vi "LV_call_transfer.vi"() -> ()   [LabVIEW 2020]
panel:
  out "return code":i32
  out "standard output":string
  out "error out":errorcluster
  out "Path to Python script":path
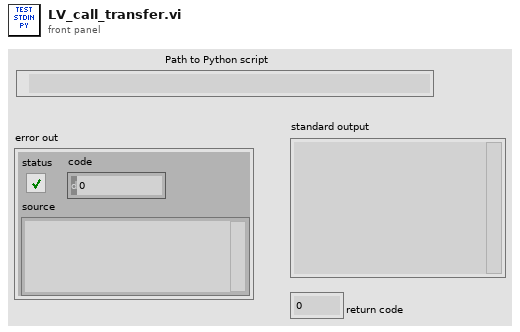
[diagram p1: front panel]
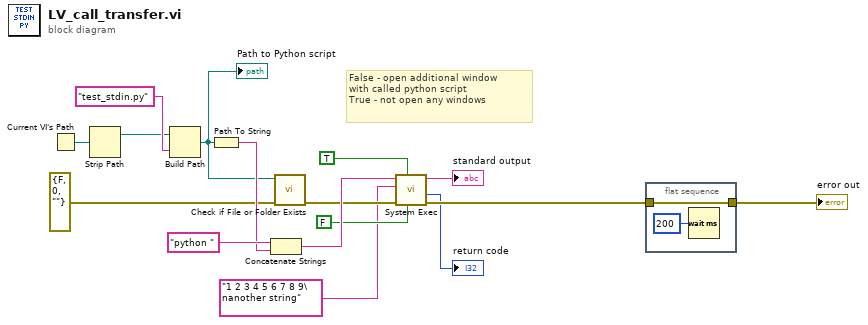
[diagram p0: block diagram]
diagram:
  # "False - open additional window\nwith called python script\nTrue - not open any windows"
  n1 = Current VI's Path() -> (path=w16:path)
  n2 = Strip Path(path=w16) -> (stripped path=w10:path)  [unwired: 1 out]
  n3 = Build Path(base path=w10, name or relative path="test_stdin.py" ("string")) -> (appended path=w8:path)
  "Path to Python script" <- w8
  n4 = Path To String(path=w8) -> (string=w11:string)
  n5 = Concatenate Strings("python " ("command line"), w11) -> (w14:string)
  n6 = call <vilib>:"Check if File or Folder Exists.vi"("error in (no error)"=errorcluster {"status"=FALSE, "code"=0, "source"=""}, "path"=w8) -> ("error out"=w7:errorcluster)  [unwired: 7 in, 2 out]
  n7 = call <vilib>:"System Exec.vi"("run minimized? (F)"=FALSE, "wait until completion? (T)"=TRUE, "error in (no error)"=w7, "standard input"="1 2 3 4 5 6 7 8 9\nanother string", "command line"=w14) -> ("error out"=w4:errorcluster, "return code"=→"return code":i32, "standard output"=→"standard output":string)  [unwired: 3 in, 1 out]
  n8 = flat-sequence {
    tunnel: w4 -> [w17]
    tunnel: [w17] -> w3
    frame #0 {
      n9 = Wait (ms)(milliseconds to wait=u32 200) -> ()  [unwired: 1 out]
    }
  }
  "error out" <- w3
